vi "公式节点.vi"() -> ()   [LabVIEW 2020]
doc: "本VI是为《我和LabVIEW》一书编写的示例。\n关于本书的介绍请参考网页：\nhttp://ruanqizhen.spaces.live.com/blog/cns!5852D4F797C53FB6!4310.entry"
uses:
  <vilib>/express/express arith-compare/Formula/XNode/ExpressFormulaBlockNode.xnode
panel:
  out "结果":dbl
  in  "a":i32
  out "y":i32
  in  "x":i32
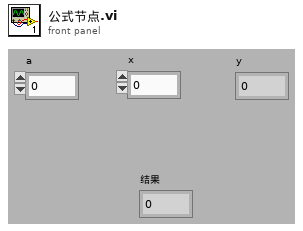
[diagram p1: front panel]
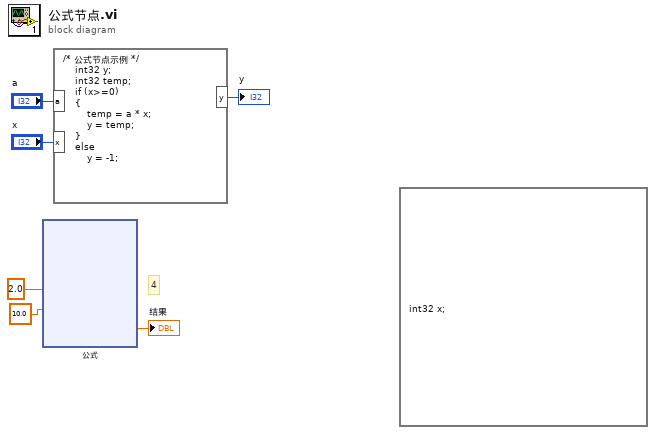
[diagram p0: block diagram]
diagram:
  # "4"
  n1 = xnode "公式"("X1"=2.0, "X2"=10.0) -> ("结果"=→"结果":dbl)  [unwired: 1 in, 1 out]
  n2 = formula code="/* 公式节点示例 */\n    int32 y;\n    int32 temp;\n    if (x>=0)\n    {\n        temp = a * x;\n        y = temp;\n    }\n    else\n        y = -1;"("x"="x", "a"="a") -> ("y"=→"y":i32)
  n3 = formula code="int32 x;"() -> ()
